vi "TypeDefAssessmentInfo.vi"() -> ()   [LabVIEW 2019]
uses:
  TypeDefAssessmentInfo.ctl
  All_In_One/States/Assessment_Modes.ctl
panel:
  out "?":T1
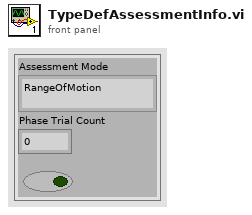
[diagram p1: front panel]
types:
  T1 = typedef "TypeDefAssessmentInfo.ctl" = cluster{"Assessment Mode":T2, "Phase Trial Count":i16, "Left Hand":bool}
  T2 = typedef "Assessment_Modes.ctl" = enum8{"RangeOfMotion", "Force", "Motor", "Sensorimotor", "PositionMatching", "PreciseReaching"}
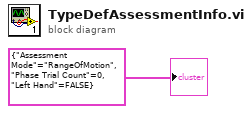
[diagram p0: block diagram]
diagram:
  "?" <- T1 {"Assessment Mode"=enum."RangeOfMotion", "Phase Trial Count"=0, "Left Hand"=FALSE}
